vi "camera-read_exposure-auto.vi"(0 "IMAQ Session In":refnum<k11>, 5 "error in (no error)":errorcluster) -> (14 "IMAQ Session Out":refnum<k11>, 15 "Option":string, 16 "Address":string, 18 "Data Read":string, 19 "error out":errorcluster)   [LabVIEW 2012]
panel:
  out "Loop Iteration":i32
  out "ACK/NAK":string
  out "String to Write":string
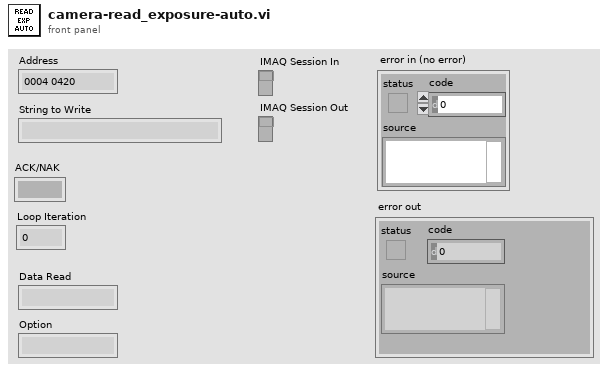
[diagram p1: front panel]
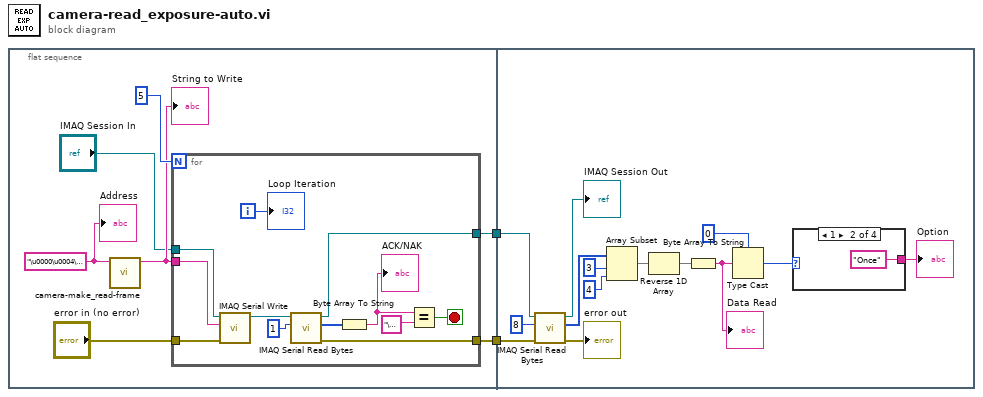
[diagram p0: block diagram]
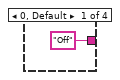
[diagram p2: hidden frame]
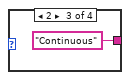
[diagram p3: hidden frame]
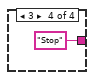
[diagram p4: hidden frame]
diagram:
  n1 = flat-sequence {
    tunnel: [w8] -> w2
    tunnel: [w7] -> w1
    tunnel: w2 -> [w34]
    tunnel: w1 -> [w33]
    frame #0 {
      w6 = "\u0000\u0004\u0004 " ("Address")
      n2 = call "camera-make_read-frame.vi"("Address"=w6) -> ("Serial String"=w5:string)  [unwired: 10 in]
      "String to Write" <- w5
      n3 = for {
        N: 5 -> [_]
        tunnel: "IMAQ Session In" -> [w21]
        tunnel: w5 -> [w20]
        tunnel: [w13] -> w8
        tunnel: "error in (no error)" -> [w19]
        tunnel: [w12] -> w7
        i -> [w16]
        stop <- w18 stop-if-true
        n4 = call <vilib>:"IMAQ Serial Write.vi"("error in (no error)"=w19, "String to write"=w20, "IMAQ Session In"=w21) -> ("IMAQ Session Out"=w14:refnum<k11>)  [unwired: 5 in, 1 out]
        n5 = call <vilib>:"IMAQ Serial Read Bytes.vi"("Bytes to Read"=u32 1, "IMAQ Session In"=w14) -> ("error out"=w12:errorcluster, "Byte Array"=w11:i8[], "IMAQ Session Out"=w13:refnum<k11>)  [unwired: 4 in, 1 out]
        n6 = Byte Array To String(unsigned byte array=w11) -> (string=w10:string)
        "ACK/NAK" <- w10
        n7 = Equal?(x=w10, y="\u0006") -> (x = y?=w18:bool)
        "Loop Iteration" <- w16
      }
      "Address" <- w6
    }
    frame #1 {
      n8 = call <vilib>:"IMAQ Serial Read Bytes.vi"("error in (no error)"=w33, "Bytes to Read"=u32 8, "IMAQ Session In"=w34) -> ("error out"=→"error out":errorcluster, "Byte Array"=w22:i8[], "IMAQ Session Out"=→"IMAQ Session Out":refnum<k11>)  [unwired: 3 in, 1 out]
      n9 = Array Subset(array=w22, index=3, length=4) -> (w28:i8[])
      n10 = Reverse 1D Array(array=w28) -> (reversed array=w27:i8[])
      n11 = Byte Array To String(unsigned byte array=w27) -> (string=w26:string)
      "Data Read" <- w26
      n12 = Type Cast(type=0, x=w26) -> (*(type *) &x=w24:i32)
      n13 = case shown="1" w24 {
        tunnel: ["Off" "Once" "Continuous" "Stop"] -> w23
        frame 0, Default {
        }
        frame 1 {
        }
        frame 2 {
        }
        frame 3 {
        }
      }
      "Option" <- w23
    }
  }
